vi "t1-t.vi"() -> ()   [LabVIEW 2014]
uses:
  <vilib>/regexp/Match Regular Expression.xnode
  <vilib>/FTP/NI_FTP.lvlib
panel:
  out "일치 구문 앞":string
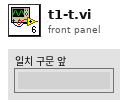
[diagram p1: front panel]
types:
  T1 = typedef "NI_FTP.lvlib/FTP Session.ctl" = refnum<k5>
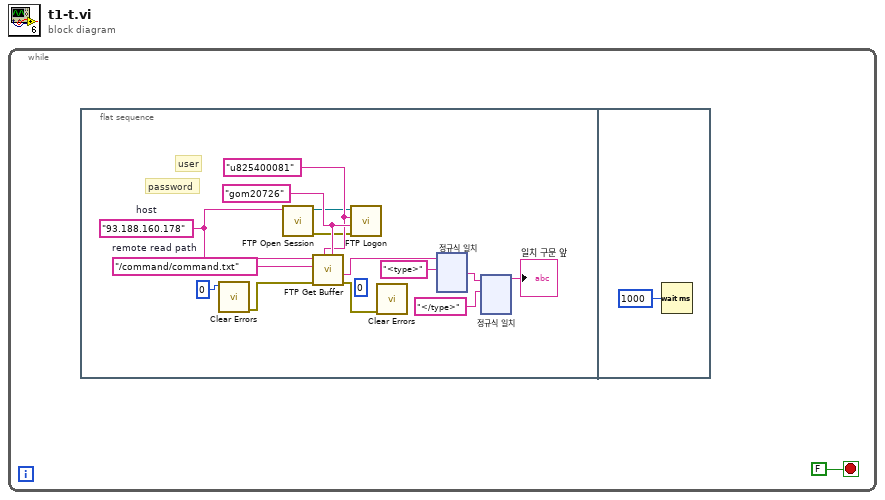
[diagram p0: block diagram]
diagram:
  n1 = while {
    stop <- FALSE stop-if-true
    n2 = flat-sequence {
      frame #0 {
        (unwired) 0 ("specific error code to clear (0: all)")
        w6 = "gom20726"
        w5 = "u825400081"
        w8 = "/command/command.txt"  # remote read path
        w7 = "93.188.160.178"  # host
        # "user"
        # "password"
        n3 = call <vilib>:"Clear Errors.vi"("specific error code to clear (0: all)"=0) -> ("error out"=w9:errorcluster)  [unwired: 5 in, 1 out]
        n4 = call <vilib>:"FTP Open Session.vi"("address"=w7) -> ("error out"=w4:errorcluster, "ftp session"=w3:T1)  [unwired: 7 in, 2 out]
        n5 = call <vilib>:"FTP Get Buffer.vi"("password"=w6, "user"=w5, "error in (no error)"=w9, "remote path"=w8, "host"=w7) -> ("error out"=w11:errorcluster, "data"=w12:string)  [unwired: 4 in, 1 out]
        n6 = call <vilib>:"FTP Logon.vi"("error in (no error)"=w4, "password"=w6, "user"=w5, "ftp session"=w3) -> ()  [unwired: 4 in, 4 out]
        n7 = call <vilib>:"Clear Errors.vi"("error in (no error)"=w11) -> ()  [unwired: 5 in, 2 out]
        n8 = xnode "정규식 일치"("입력 문자열"=w12, "정규식"="<type>") -> ("일치 구문 뒤"=w14:string)  [unwired: 4 in, 4 out]
        n9 = xnode "정규식 일치"("입력 문자열"=w14, "정규식"="</type>") -> ("일치 구문 앞"=→"일치 구문 앞":string)  [unwired: 4 in, 4 out]
      }
      frame #1 {
        n10 = Wait (ms)(milliseconds to wait=u32 1000 ("대기 시간(ms)")) -> ()  [unwired: 1 out]
      }
    }
  }
